vi "SSS_V1.1(TEST).vi"() -> ()   [LabVIEW 2017]
uses:
  <vilib>/measure/maspectr.llb/Power Spectrum and PSD Export Mode.ctl
  <vilib>/DAQmx/write.llb/DAQmx Write (Analog Wfm 1Chan NSamp).vi
  <vilib>/DAQmx/read.llb/DAQmx Read (Analog 1D Wfm NChan NSamp).vi
  <vilib>/DAQmx/create/channels.llb/DAQmx Create Channel (AI-Voltage-Basic).vi
  <vilib>/DAQmx/configure/timing.llb/DAQmx Timing (Sample Clock).vi
  <vilib>/DAQmx/create/channels.llb/DAQmx Create Channel (AO-Voltage-Basic).vi
  <vilib>/measure/maspectr.llb/FFT Power Spectrum and PSD for 1 Chan.vi
  <vilib>/DAQmx/miscellaneous.llb/DAQmx Fill In Error Info.vi
  <vilib>/Analysis/3filter.llb/FIR Filter (DBL).vi
  <vilib>/Analysis/NI_AALBase.lvlib
  <vilib>/measure/NI_MAPro.lvlib
panel:
  out "원소":sgl
  out "크기":i32
  in  "정지":bool
  out "Pack(4byte)":string
  out "TX Spectrum":cluster{"f0":dbl, "df":dbl, "magnitude":dbl[]}(graph)
  out "TX Signal":waveform(dbl)(graph)
  out "Signal Processing Result":waveform(dbl)(graph)
  in  "송신 채널 설정":tag="Dev3/ao0"
  in  "송신 디바이스 이름":tag="Dev3"
  in  "Pulse length(sec)":dbl=0.0004 format="%#_6p"
  in  "Stop Frequency(Hz)":dbl=470000.0 format="%#_6p"
  in  "Start Frequency(Hz)":dbl=430000.0 format="%#_6p"
  in  "Number of Sample":i32=150000
  out "RX.CH2":waveform(dbl)(graph)
  out "RX.CH1":waveform(dbl)(graph)
  in  "RX Time(sec)":dbl=2.0
  in  "수신 디바이스 이름":tag="Dev3"
  in  "수신 채널 설정":tag="Dev3/ai0:1"
  in  "sampling rate":dbl=1500000.0 caption="Sampling Frequency" format="%0.2f"
  in  "sample mode":i32(ring)=10123 caption="샘플 모드" items=["유한 샘플"=10178, "연속 샘플"=10123, "하드웨어 타이밍에 의한 단일 포인트"=12522]
  # "TX Variable Setting"
  # "ADC/DAC Setting"
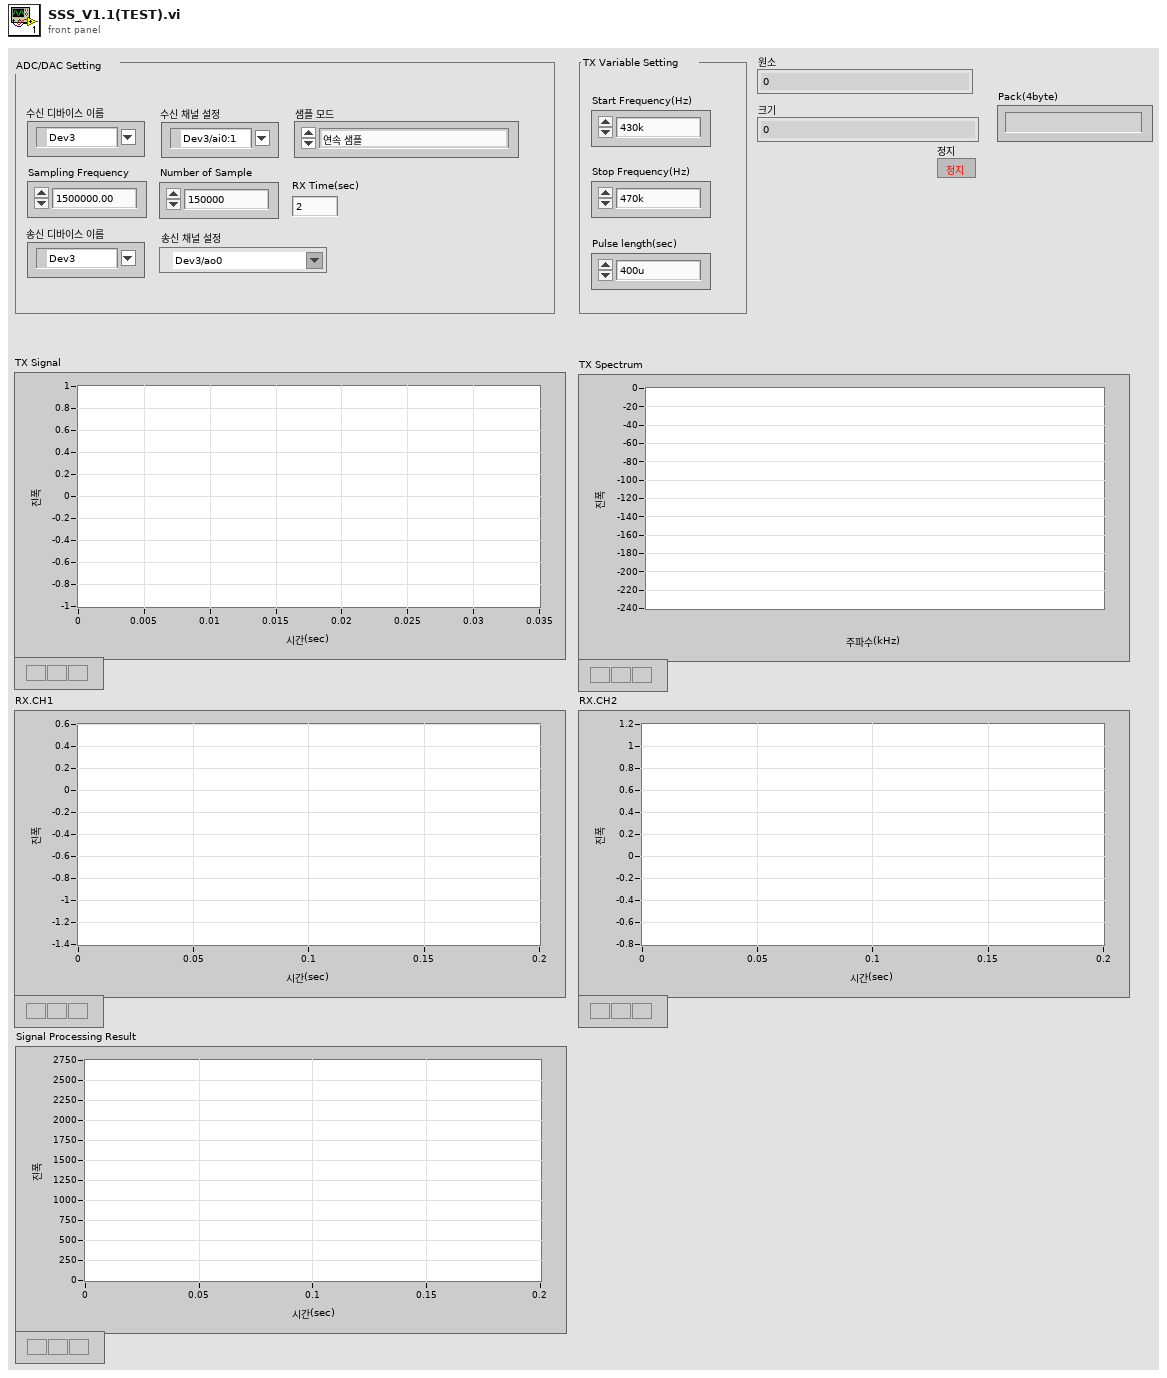
[diagram p1: front panel]
types:
  T1 = typedef "NI_MAPro.lvlib/Power Spectrum and PSD Export Mode.ctl" = u16
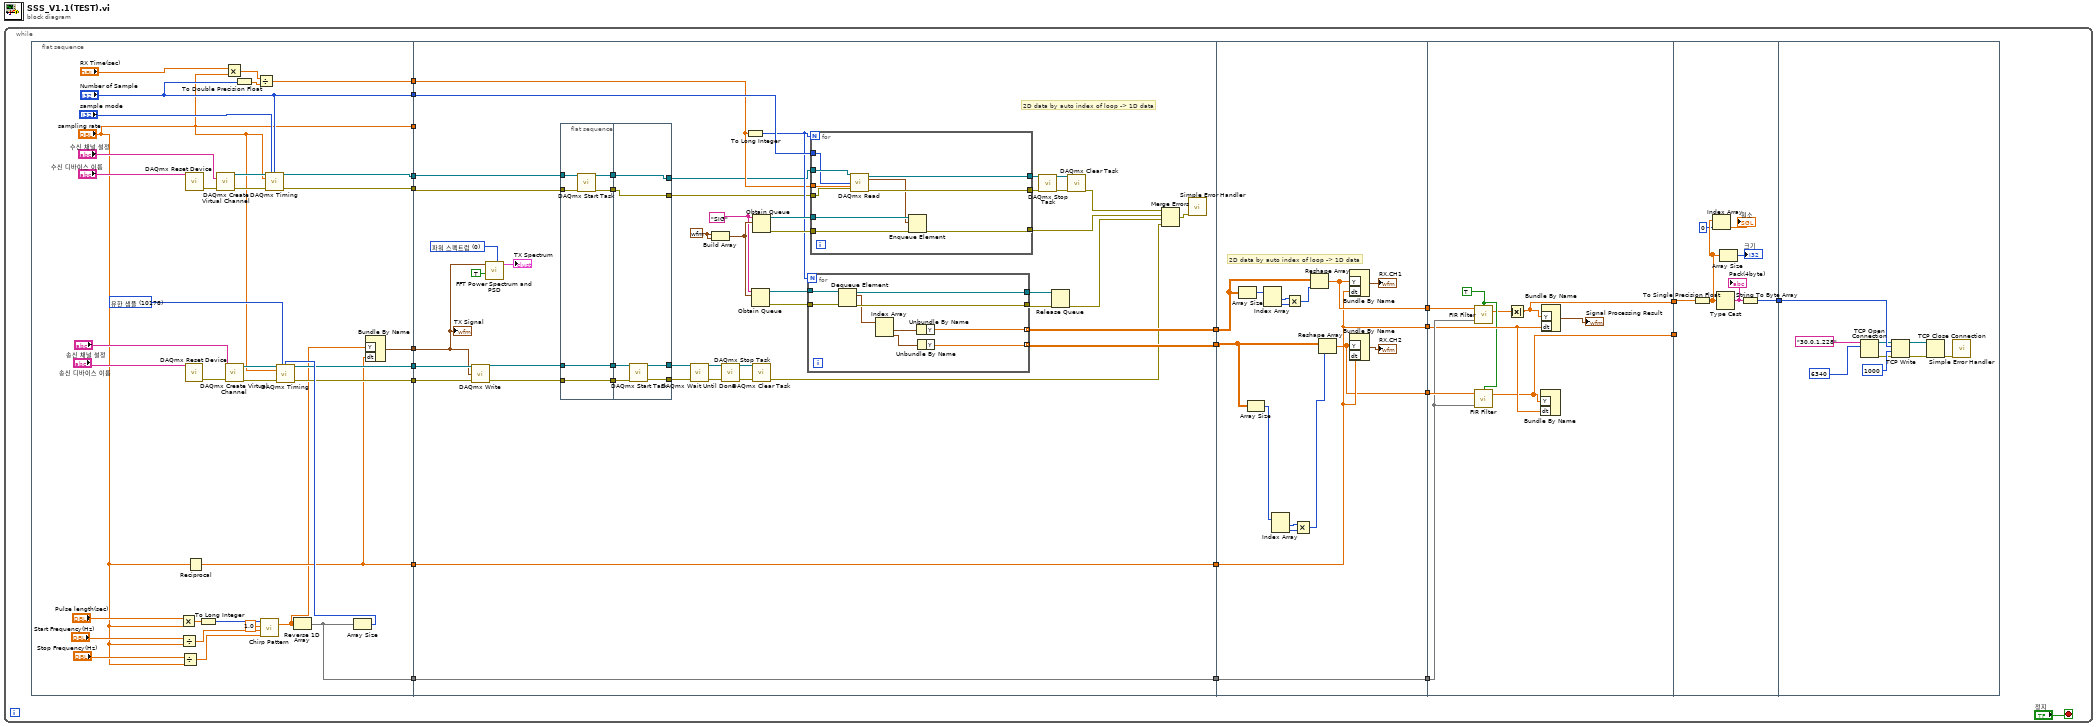
[diagram p0: block diagram]
diagram:
  n1 = while {
    stop <- "정지" stop-if-true
    n2 = flat-sequence {
      tunnel: ["sampling rate"] -> w22
      tunnel: ["Number of Sample"] -> w21
      tunnel: [w47] -> w20
      tunnel: [w46] -> w19
      tunnel: [w45] -> w18
      tunnel: [w27] -> w17
      tunnel: [w30] -> w16
      tunnel: [w29] -> w15
      tunnel: [w26] -> w14
      tunnel: [w24] -> w13
      tunnel: w22 -> [_]
      tunnel: w21 -> [w91]
      tunnel: w20 -> [w77]
      tunnel: w19 -> [w82]
      tunnel: w18 -> [w89]
      tunnel: [w84] -> w12
      tunnel: [w83] -> w11
      tunnel: w17 -> [w58]
      tunnel: [w58] -> w10
      tunnel: w16 -> [w76]
      tunnel: w15 -> [w75]
      tunnel: w14 -> [w62]
      tunnel: w13 -> [w63]
      tunnel: [w63] -> w9
      tunnel: w12 -> [w147]
      tunnel: w11 -> [w142]
      tunnel: w10 -> [w138]
      tunnel: [w140] -> w8
      tunnel: w9 -> [w139]
      tunnel: [w139] -> w7
      tunnel: [w138] -> w6
      tunnel: [w137] -> w5
      tunnel: w8 -> [w160]
      tunnel: w7 -> [w157]
      tunnel: w6 -> [w156]
      tunnel: w5 -> [w158]
      tunnel: [w153] -> w4
      tunnel: [w154] -> w3
      tunnel: w4 -> [w165]
      tunnel: w3 -> [_]
      tunnel: [w166] -> w2
      tunnel: w2 -> [w174]
      frame #0 {
        w33 = 10178 items=["유한 샘플"=10178, "연속 샘플"=10123, "하드웨어 타이밍에 의한 단일 포인트"=12522] ("sample mode")
        n3 = Multiply(x="Pulse length(sec)", y="sampling rate") -> (x*y=w43:dbl)
        n4 = Divide(x="Start Frequency(Hz)", y="sampling rate") -> (x/y=w40:dbl)
        n5 = Divide(x="Stop Frequency(Hz)", y="sampling rate") -> (x/y=w37:dbl)
        n6 = call <vilib>:"DAQmx Reset Device.vi"("device in"="송신 디바이스 이름") -> ("error out"=w36:errorcluster)  [unwired: 1 in, 13 out]
        n7 = call <vilib>:"DAQmx Reset Device.vi"("device in"="수신 디바이스 이름") -> ("error out"=w51:errorcluster)  [unwired: 1 in, 13 out]
        n8 = Reciprocal(x="sampling rate") -> (1/x=w27:dbl)
        n9 = To Long Integer(number=w43) -> (32bit integer=w42:i32)
        n10 = call-poly <vilib>:"DAQmx Create Virtual Channel.vi"("physical channels"="수신 채널 설정", "error in"=w51) -> ("task out"=w50:refnum<k21>, "error out"=w49:errorcluster)  [unwired: 7 in, 5 out]
        n11 = Multiply(x="RX Time(sec)", y="sampling rate") -> (x*y=w54:dbl)
        n12 = call-poly <vilib>:"DAQmx Create Virtual Channel.vi"("physical channels"="송신 채널 설정", "error in"=w36) -> ("task out"=w32:refnum<k21>, "error out"=w35:errorcluster)  [unwired: 7 in, 5 out]
        n13 = To Double Precision Float(number="Number of Sample") -> (double precision float=w55:dbl)
        n14 = Divide(x=w54, y=w55) -> (x/y=w45:dbl)
        n15 = call <vilib>:"Chirp Pattern.vi"("f2"=w37, "f1"=w40, "amplitude"=1.0, "samples"=w42) -> ("Chirp Pattern"=w23:dbl[])  [unwired: 1 out]
        n16 = call-poly <vilib>:"DAQmx Timing.vi"("task/channels in"=w50, "sample mode"="sample mode", "samples per channel"="Number of Sample", "rate"="sampling rate", "error in"=w49) -> ("task out"=w47:refnum<k21>, "error out"=w46:errorcluster)  [unwired: 2 in, 7 out]
        n17 = Reverse 1D Array(array=w23) -> (reversed array=w24:dbl[])
        n18 = Array Size(array=w24) -> (size(s)=w34:i32)
        n19 = call-poly <vilib>:"DAQmx Timing.vi"("task/channels in"=w32, "sample mode"=w33, "samples per channel"=w34, "rate"="sampling rate", "error in"=w35) -> ("task out"=w30:refnum<k21>, "error out"=w29:errorcluster)  [unwired: 2 in, 7 out]
        n20 = Bundle By Name("Y"=w23, "dt"=w27) -> (w26:waveform(dbl))  [unwired: 1 in]
      }
      frame #1 {
        w60 = T1 0 items=["파워 스펙트럼", "파워 스펙트럼 밀도"] ("export mode")
        w88 = "SIG" ("이름(이름없음)")
        w93 = waveform(dbl) {"t0"=timestamp(0 s since 1904-01-01), "dt"=1.0, "Y"=[]} ("Waveform")
        # "2D data by auto index of loop -> 1D data"
        n21 = call-poly <vilib>:"DAQmx Write.vi"("task/channels in"=w76, "data"=w62, "error in"=w75) -> ("task out"=w72:refnum<k21>, "error out"=w74:errorcluster)  [unwired: 10 in, 1 out]
        n22 = call-poly <vilib>:"FFT Power Spectrum and PSD.vi"("export mode"=w60, "dB On (F)"=TRUE, "time signal"=w62) -> ("Power Spectrum / PSD"=→"TX Spectrum":cluster{"f0":dbl, "df":dbl, "magnitude":dbl[]})  [unwired: 5 in, 3 out]
        n23 = flat-sequence {
          tunnel: w82 -> [w110]
          tunnel: [w109] -> w81
          tunnel: [w108] -> w78
          tunnel: w77 -> [w107]
          tunnel: w74 -> [w106]
          tunnel: [w106] -> w73
          tunnel: w72 -> [w105]
          tunnel: [w105] -> w71
          tunnel: w81 -> [w116]
          tunnel: [w116] -> w80
          tunnel: [w115] -> w79
          tunnel: w78 -> [w115]
          tunnel: w73 -> [w114]
          tunnel: w71 -> [w113]
          tunnel: [w112] -> w66
          tunnel: [w111] -> w65
          frame #0 {
            n24 = call <vilib>:"DAQmx Start Task.vi"("task/channels in"=w107, "error in"=w110) -> ("task out"=w108:refnum<k21>, "error out"=w109:errorcluster)  [unwired: 12 in]
          }
          frame #1 {
            n25 = call <vilib>:"DAQmx Start Task.vi"("task/channels in"=w113, "error in"=w114) -> ("task out"=w112:refnum<k21>, "error out"=w111:errorcluster)  [unwired: 12 in]
          }
        }
        n26 = call <vilib>:"DAQmx Wait Until Done.vi"("task/channels in"=w66, "error in"=w65) -> ("task out"=w68:refnum<k21>, "error out"=w67:errorcluster)  [unwired: 12 in]
        n27 = Build Array(w93, w93) -> (w92:waveform(dbl)[])
        n28 = call <vilib>:"DAQmx Stop Task.vi"("task/channels in"=w68, "error in"=w67) -> ("task out"=w70:refnum<k21>, "error out"=w69:errorcluster)  [unwired: 12 in]
        n29 = To Long Integer(number=w89) -> (32bit integer=w90:i32)
        n30 = Obtain Queue(name (unnamed)=w88, element data type=w92) -> (queue out=w96:refnum<queue>, error out=w95:errorcluster)  [unwired: 3 in, 1 out]
        n31 = Obtain Queue(name (unnamed)=w88, element data type=w92) -> (queue out=w102:refnum<queue>, error out=w101:errorcluster)  [unwired: 3 in, 1 out]
        n32 = call <vilib>:"DAQmx Clear Task.vi"("task in"=w70, "error in"=w69) -> ("error out"=w64:errorcluster)  [unwired: 13 in]
        n33 = for {
          N: w90 -> [_]
          tunnel: w96 -> [w125]
          tunnel: w95 -> [w124]
          tunnel: [w123] -> w87
          tunnel: [w121] -> w85
          tunnel: [w118] -> w84 mode=indexing
          tunnel: [w119] -> w83 mode=indexing
          n34 = Dequeue Element(queue=w125, error in (no error)=w124) -> (queue out=w121:refnum<queue>, element=w122:waveform(dbl)[], error out=w123:errorcluster)  [unwired: 1 in, 1 out]
          n35 = Index Array(array=w122) -> (element #1=w120:waveform(dbl), element #2=w117:waveform(dbl))  [unwired: 2 in]
          n36 = Unbundle By Name(w120) -> ("Y"=w118:dbl[])
          n37 = Unbundle By Name(w117) -> ("Y"=w119:dbl[])
        }
        n38 = for {
          N: w90 -> [_]
          tunnel: w102 -> [w135]
          tunnel: w101 -> [w134]
          tunnel: [w133] -> w99
          tunnel: [w132] -> w98
          tunnel: [w131] -> w97
          tunnel: w79 -> [w129]
          tunnel: w80 -> [w128]
          tunnel: w91 -> [w127]
          tunnel: w89 -> [w126]
          n39 = call-poly <vilib>:"DAQmx Read.vi"("task/channels in"=w129, "number of samples per channel"=w127, "timeout"=w126, "error in"=w128) -> ("task out"=w132:refnum<k21>, "data"=w130:waveform(dbl)[], "error out"=w131:errorcluster)  [unwired: 9 out]
          n40 = Enqueue Element(queue=w135, element=w130, error in (no error)=w134) -> (error out=w133:errorcluster)  [unwired: 1 in, 2 out]
        }
        n41 = call <vilib>:"DAQmx Stop Task.vi"("task/channels in"=w98, "error in"=w97) -> ("task out"=w103:refnum<k21>, "error out"=w104:errorcluster)  [unwired: 12 out]
        n42 = Release Queue(queue=w85, error in (no error)=w87) -> (error out=w86:errorcluster)  [unwired: 3 out]
        n43 = call <vilib>:"DAQmx Clear Task.vi"("task in"=w103, "error in"=w104) -> ("error out"=w100:errorcluster)  [unwired: 13 out]
        n44 = Merge Errors(w100, w99, w86, w64) -> (w94:errorcluster)
        n45 = call <vilib>:"Simple Error Handler.vi"("error in (no error)"=w94) -> ()  [unwired: 4 in, 5 out]
        "TX Signal" <- w62
      }
      frame #2 {
        # "2D data by auto index of loop -> 1D data"
        n46 = Array Size(array=w147) -> (size(s)=w148:i32[])
        n47 = Array Size(array=w142) -> (size(s)=w143:i32[])
        n48 = Index Array(array=w148) -> (element #1=w150:i32, element #2=w149:i32)  [unwired: 2 in]
        n49 = Index Array(array=w143) -> (element #1=w145:i32, element #2=w144:i32)  [unwired: 2 in]
        n50 = Multiply(x=w150, y=w149) -> (x*y=w151:i32)
        n51 = Multiply(x=w145, y=w144) -> (x*y=w146:i32)
        n52 = Reshape Array(w147, w151) -> (w140:dbl[])
        n53 = Reshape Array(w142, w146) -> (w137:dbl[])
        n54 = Bundle By Name("Y"=w140, "dt"=w138) -> (→"RX.CH1":waveform(dbl))  [unwired: 1 in]
        n55 = Bundle By Name("Y"=w137, "dt"=w138) -> (→"RX.CH2":waveform(dbl))  [unwired: 1 in]
      }
      frame #3 {
        w155 = TRUE ("init/cont (init:F)")
        n56 = call-poly <vilib>:"FIR Filter.vi"("init/cont (init:F)"=w155, "FIR Coefficients"=w157, "X"=w158) -> ("Filtered X"=w154:dbl[])  [unwired: 1 in, 1 out]
        n57 = call-poly <vilib>:"FIR Filter.vi"("init/cont (init:F)"=w155, "FIR Coefficients"=w157, "X"=w160) -> ("Filtered X"=w152:dbl[])  [unwired: 1 in, 1 out]
        n58 = Absolute Value(x=w152) -> (abs(x)=w153:dbl[])
        n59 = Bundle By Name("Y"=w154, "dt"=w156) -> ()  [unwired: 1 in, 1 out]
        n60 = Bundle By Name("Y"=w153, "dt"=w156) -> (→"Signal Processing Result":waveform(dbl))  [unwired: 1 in]
      }
      frame #4 {
        n61 = To Single Precision Float(number=w165) -> (single precision float=w163:sgl[])
        n62 = Index Array(array=w163, index=0 ("인덱스")) -> (element=→"원소":sgl)
        n63 = Type Cast(x=w163) -> (*(type *) &x=w167:string)  [unwired: 1 in]
        "Pack(4byte)" <- w167
        n64 = Array Size(array=w163) -> (size(s)=→"크기":i32)
        n65 = String To Byte Array(string=w167) -> (unsigned byte array=w166:u8[])
      }
      frame #5 {
        n66 = TCP Open Connection(address="30.0.1.228" ("주소"), remote port or service name=u16 6340 ("원격 포트 또는 서비스 이름")) -> (connection ID=w171:refnum<k5>, error out=w170:errorcluster)  [unwired: 3 in]
        n67 = TCP Write(connection ID=w171, data in=w174, error in (no error)=w170, 9:1000 ("타임아웃 ms (25000)")) -> (connection ID out=w176:refnum<k5>, error out=w175:errorcluster)  [unwired: 1 out]
        n68 = TCP Close Connection(connection ID=w176, error in (no error)=w175) -> (error out=w173:errorcluster)  [unwired: 1 in, 1 out]
        n69 = call <vilib>:"Simple Error Handler.vi"("error in (no error)"=w173) -> ()  [unwired: 4 in, 5 out]
      }
    }
  }
